vi "filter_dynamic.vi"() -> ()   [LabVIEW 2017]
panel:
  out "Waveform Chart":dynamicdata(graph)
  in  "stop":bool
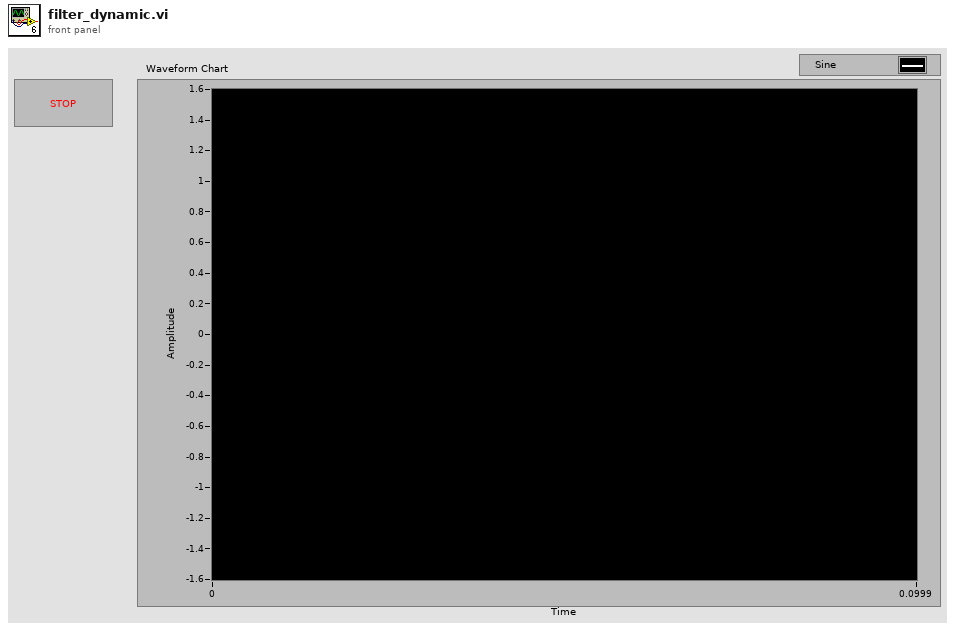
[diagram p1: front panel]
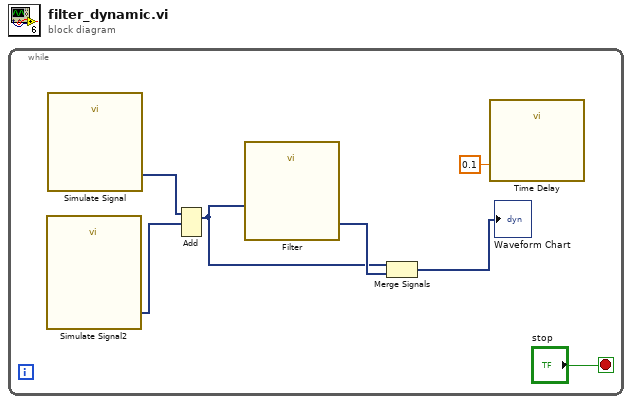
[diagram p0: block diagram]
diagram:
  n1 = while {
    stop <- "stop" stop-if-true
    n2 = call "Simulate Signal2"() -> ("Sine"=w5:dynamicdata)  [unwired: 14 in, 1 out]
    n3 = call "Simulate Signal"() -> ("Sine"=w6:dynamicdata)  [unwired: 14 in, 1 out]
    n4 = Add(1:w5, 2:w6) -> (0:w4:dynamicdata)  [unwired: 1 in, 1 out]
    n5 = call "Filter"("Signal"=w4) -> ("Filtered Signal"=w7:dynamicdata)  [unwired: 9 in, 1 out]
    n6 = Merge Signals(w4, w7) -> (→"Waveform Chart":dynamicdata)
    n7 = call "Time Delay"("Delay Time (s)"=0.1) -> ()  [unwired: 10 in, 1 out]
  }
